vi "SHA256 Hash.vi"(8 "error in (no error)":errorcluster, 11 "string to hash":string) -> (0 "error out":errorcluster, 2 "hash bytes":u8[](array[numeric]) format="%02x", 3 "hex string hash":string)   [LabVIEW 2013]
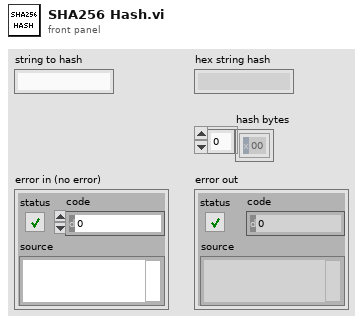
[diagram p1: front panel]
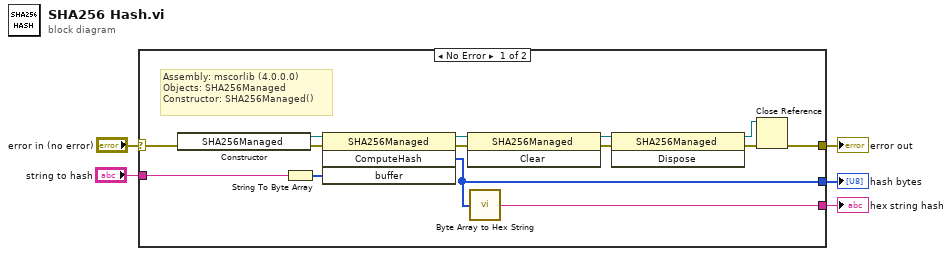
[diagram p0: block diagram]
diagram:
  n1 = case shown="No Error" "error in (no error)" {
    selector: "error in (no error)" -> [w8 w20]
    tunnel: "string to hash" -> [w17 _]
    tunnel: [w7 _] -> w4
    tunnel: [w9 w20] -> w3
    tunnel: [w6 _] -> w1
    frame No Error {
      # "Assembly: mscorlib (4.0.0.0)\nObjects: SHA256Managed\nConstructor: SHA256Managed()"
      n2 = constructor class="SHA256Managed"(error in=w8) -> (reference out=w19:refnum<k24>, error out=w18:errorcluster)  [unwired: 2 in, 1 out]
      n3 = String To Byte Array(string=w17) -> (unsigned byte array=w16:u8[])
      n4 = invoke class="SHA256Managed" method="ComputeHash"(reference=w19, error in=w18, "buffer"=w16) -> (reference out=w14:refnum<k24>, error out=w15:errorcluster, "ComputeHash"=w6:u8[])  [unwired: 1 in, 1 out]
      n5 = invoke class="SHA256Managed" method="Clear"(reference=w14, error in=w15) -> (reference out=w13:refnum<k24>, error out=w12:errorcluster)  [unwired: 1 in, 1 out]
      n6 = call "Byte Array to Hex String.vi"("bytes array"=w6) -> ("hex string"=w7:string)
      n7 = invoke class="SHA256Managed" method="Dispose"(reference=w13, error in=w12) -> (reference out=w11:refnum<k24>, error out=w10:errorcluster)  [unwired: 1 in, 1 out]
      n8 = Close Reference(reference=w11, error in (no error)=w10) -> (error out=w9:errorcluster)
    }
    frame Error {
    }
  }
  "hex string hash" <- w4
  "error out" <- w3
  "hash bytes" <- w1
